vi "GetTimestamp.vi"() -> (2 "Timestamp":u32)   [LabVIEW 2018]
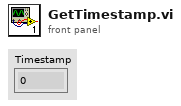
[diagram p1: front panel]
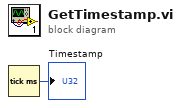
[diagram p0: block diagram]
diagram:
  n1 = Tick Count (ms)() -> (millisecond timer value=→"Timestamp":u32)
